vi "Build Path to Macro.vi"(9 "Macro Name":string, 11 "Macro Directory":path) -> (2 "Macro File Path":path)   [LabVIEW 2020, in "MacroAssert.lvlib"]
doc: "Builds the path to a macro file using the provided inputs."
uses:
  MacroAssert.lvlib
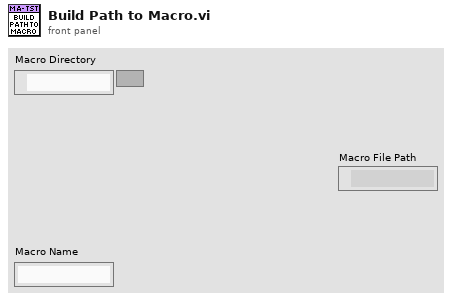
[diagram p1: front panel]
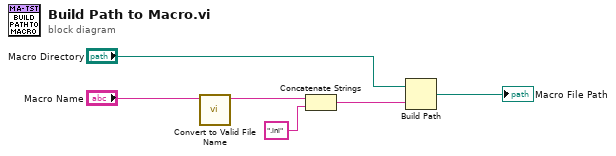
[diagram p0: block diagram]
diagram:
  n1 = call "Convert to Valid File Name.vi"("File Name"="Macro Name") -> ("Valid File Name"=w2:string)  [unwired: 9 in, 1 out]
  n2 = Concatenate Strings(w2, ".ini" ("string")) -> (w5:string)
  n3 = Build Path(base path="Macro Directory", name or relative path=w5) -> (appended path=→"Macro File Path":path)
